vi "HTML to Data Strings.vi"(11 "input string":string) -> (1 "output string":string, 2 "Cash Data String":string, 3 "Tournament Data String":string)   [LabVIEW 2021]
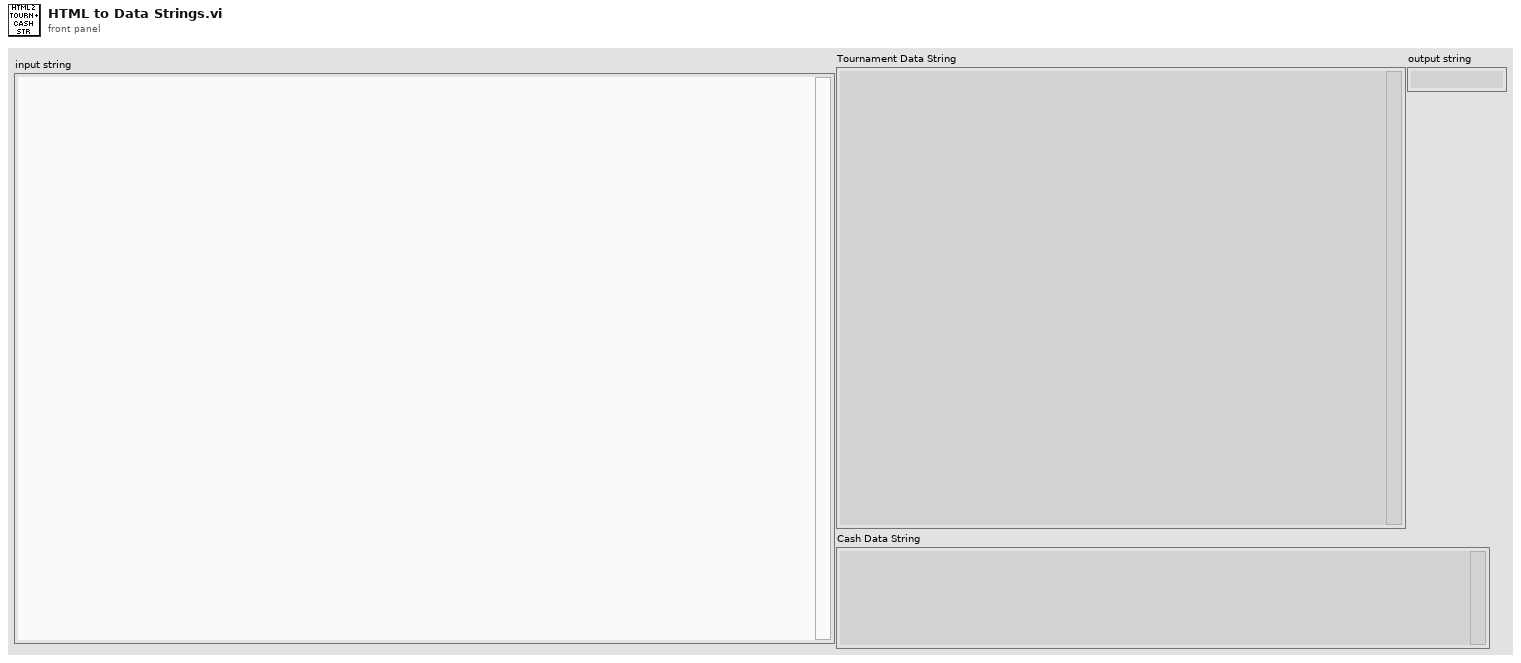
[diagram p1: front panel]
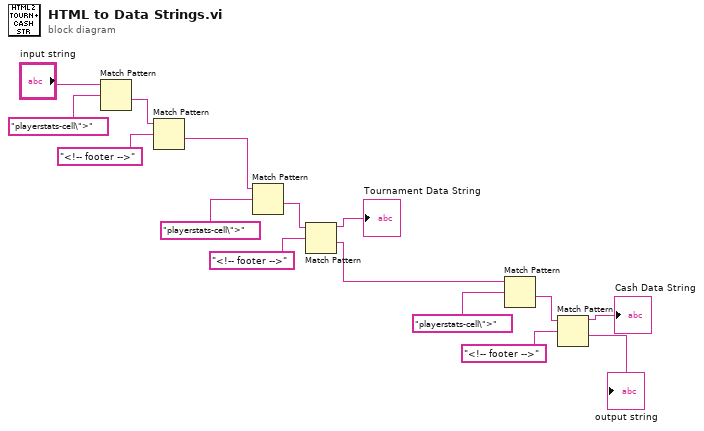
[diagram p0: block diagram]
diagram:
  n1 = Match Pattern(string="input string", regular expression="playerstats-cell\">") -> (after substring=w13:string)  [unwired: 1 in, 3 out]
  n2 = Match Pattern(string=w13, regular expression="<!-- footer -->") -> (after substring=w9:string)  [unwired: 1 in, 3 out]
  n3 = Match Pattern(string=w9, regular expression="playerstats-cell\">") -> (after substring=w11:string)  [unwired: 1 in, 3 out]
  n4 = Match Pattern(string=w11, regular expression="<!-- footer -->") -> (before substring=→"Tournament Data String":string, after substring=w4:string)  [unwired: 1 in, 2 out]
  n5 = Match Pattern(string=w4, regular expression="playerstats-cell\">") -> (after substring=w7:string)  [unwired: 1 in, 3 out]
  n6 = Match Pattern(string=w7, regular expression="<!-- footer -->") -> (before substring=→"Cash Data String":string, after substring=→"output string":string)  [unwired: 1 in, 2 out]
